vi "transport char run_subvi_08_24_12a_JW.vi"(0 "VISA session":refnum<visa-resource-name>="GPIB0::17::INSTR", 5 "Var1 sweep settings":T4={"start"=0.0, "stop"=-60.0, "step (linear only)"=-1.0, "sweep spacing (linear: 0)"=0, "sweep mode"=FALSE, "compliance (V)"=100.0, "compliance (A)"=0.001} {"compliance (A)" format="%^.2e"; "compliance (V)" format="%.2f"; "sweep spacing (linear: 0)" items=["linear", "log 10", "log 25", "log 50"]; "step (linear only)" format="%.2f"; "stop" format="%.2f"; "start" format="%.2f"}, 7 "Var2 step settings":T3={"compliance (A)"=0.001, "compliance (V)"=100.0, "start"=0.0, "total points"=7, "step"=-10.0} {"step" format="%.2f"; "start" format="%.2f"; "compliance (V)" format="%.2f"; "compliance (A)" format="%^.2e"}, 9 "integration time":u32(slide) scale=0.0..2.0, 11 "Path":path, 13 "Sample Properties:":T1 {"Date Created" format="%<%Y/%m/%d>T"}) -> (6 "graphic display":cluster{"trace":dbl[], "trace":dbl[]}(graph), 8 "Graph Cluster":cluster{"Transport":cluster{dbl[], dbl[]}[]}, 15 "error?":errorcluster)   [LabVIEW 2011]
uses:
  <vilib>/Utility/file.llb/Write To Spreadsheet File (DBL).vi
panel:
  in  "Temp (K)":dbl=100.0 format="%^.2e"
  in  "MAXIMUM":ext format="%.2e"
  in  "MINIMUM":ext=-1e-05 format="%_2e"
  out "graphic display 2":cluster{"trace":dbl[], "trace":dbl[]}(graph)
  in  "Y1 axis":string="Id"
  in  "Y2 axis settings":T2={"Y2 axis on/off"=FALSE, "MINIMUM"=-1e-07, "MAXIMUM"=1e-07, "Variable name"="", "LIN or LOG axis"=""} {"MAXIMUM" format="%.2e"; "MINIMUM" format="%.2e"}
  in  "wait time parameter":dbl=1.0
  in  "Value (Either V or A) 4":dbl
  in  "Value (Either V or A) 3":dbl
  in  "Value (Either V or A) 2":dbl
  in  "Value (V or A)":dbl
  in  "compliance (A)":dbl=0.001 format="%^.2e"
  in  "compliance (V)":dbl=100.0 format="%^.2e"
  in  "Iname":string="Is"
  in  "Vname":string="Vs"
  in  "Function":u16(ring)=4 items=["disabled", "Var1", "Var2", "Var1'", "Constant"]
  in  "Mode":u16(ring)=4 items=["V", "I", "VPulse", "IPulse", "Common"]
  in  "Iname 4":string="I4"
  in  "Vname 4":string="V4"
  in  "Function 4":u16(ring)=4 items=["disabled", "Var1", "Var2", "Var1'", "Constant"]
  in  "Mode 4":u16(ring) items=["V", "I", "VPulse", "IPulse", "Common"]
  in  "Iname 3":string="Ig"
  in  "Vname 3":string="Vg"
  in  "Function 3":u16(ring)=2 items=["disabled", "Var1", "Var2", "Var1'", "Constant"]
  in  "Mode 3":u16(ring) items=["V", "I", "VPulse", "IPulse", "Common"]
  in  "Iname 2":string="Id"
  in  "Vname 2":string="Vd"
  in  "Function 2":u16(ring)=1 items=["disabled", "Var1", "Var2", "Var1'", "Constant"]
  in  "Mode 2":u16(ring) items=["V", "I", "VPulse", "IPulse", "Common"]
  in  "reset":bool=TRUE
  # "SMU1"
  # "SMU2"
  # "SMU3"
  # "SMU4"
  # "%"
  # "nm"
  # "Device Properties:"
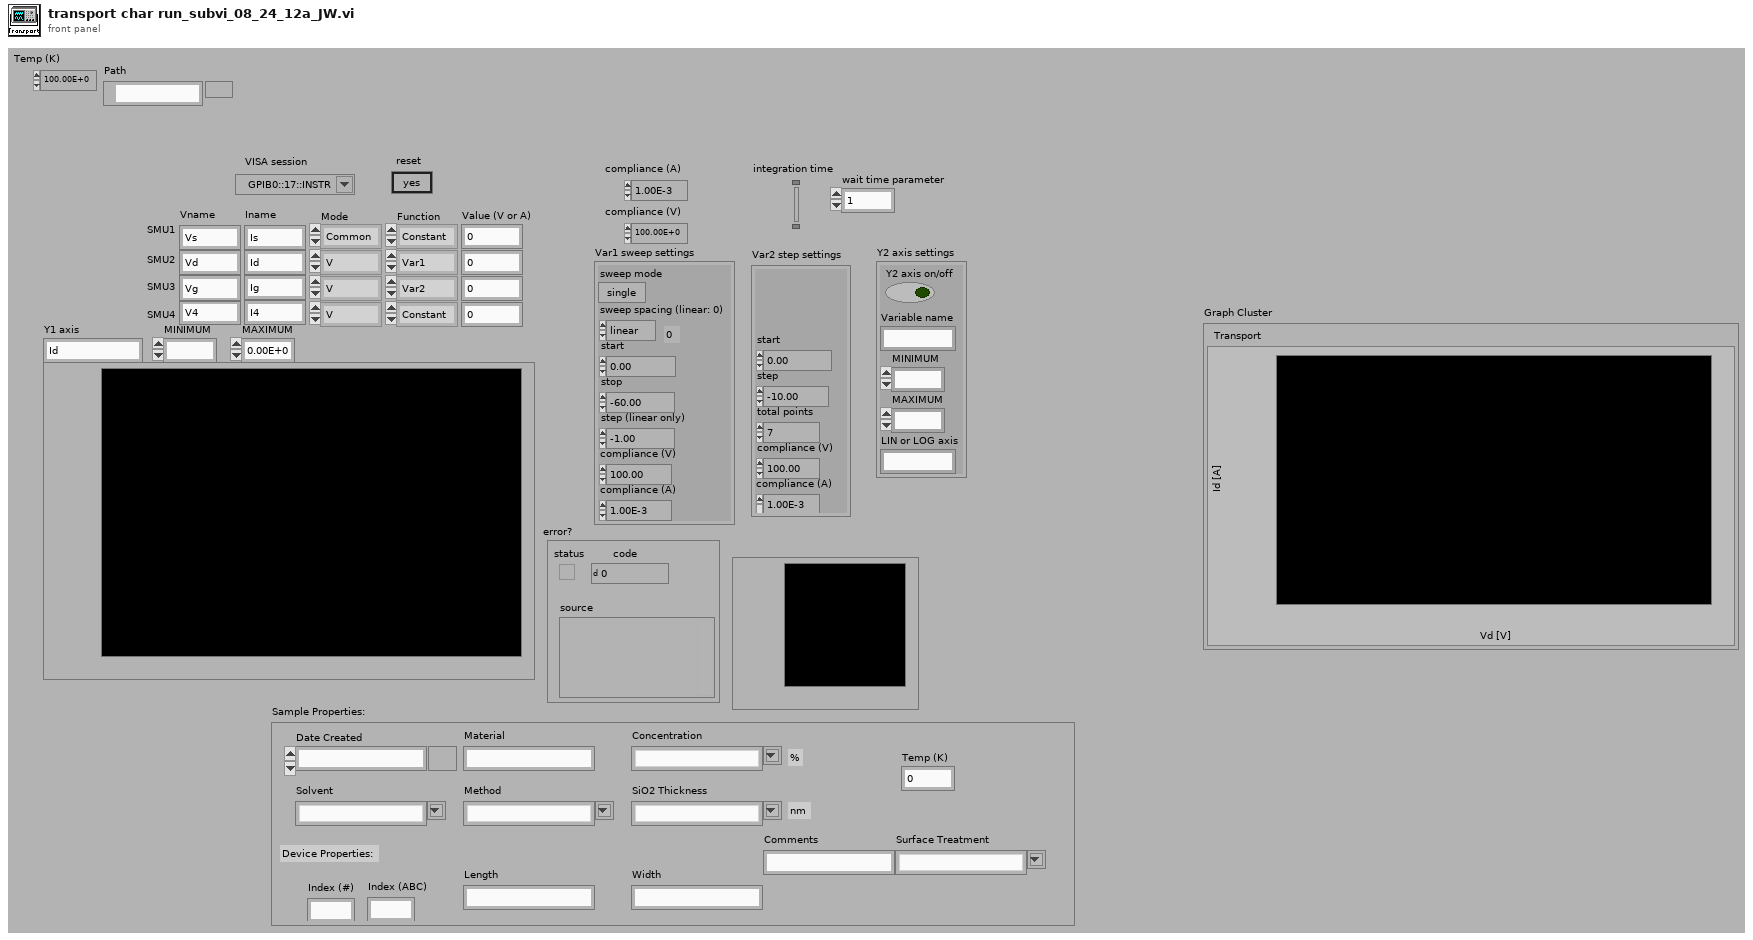
[diagram p1: front panel]
types:
  T1 = cluster{"Date Created":timestamp, "Material":string, "Solvent":string, "Concentration":string, "Method":string, "SiO2 Thickness":string, "Index (#)":string, "Index (ABC)":string, "Length":string, "Width":string, "Surface Treatment":string, "Comments":string, "Temp (K)":dbl}
  T2 = cluster{"Y2 axis on/off":bool, "MINIMUM":ext, "MAXIMUM":ext, "Variable name":string, "LIN or LOG axis":string}
  T3 = cluster{"compliance (A)":dbl, "compliance (V)":dbl, "start":dbl, "total points":u16, "step":dbl}
  T4 = cluster{"start":dbl, "stop":dbl, "step (linear only)":dbl, "sweep spacing (linear: 0)":u16, "sweep mode":bool, "compliance (V)":dbl, "compliance (A)":dbl}
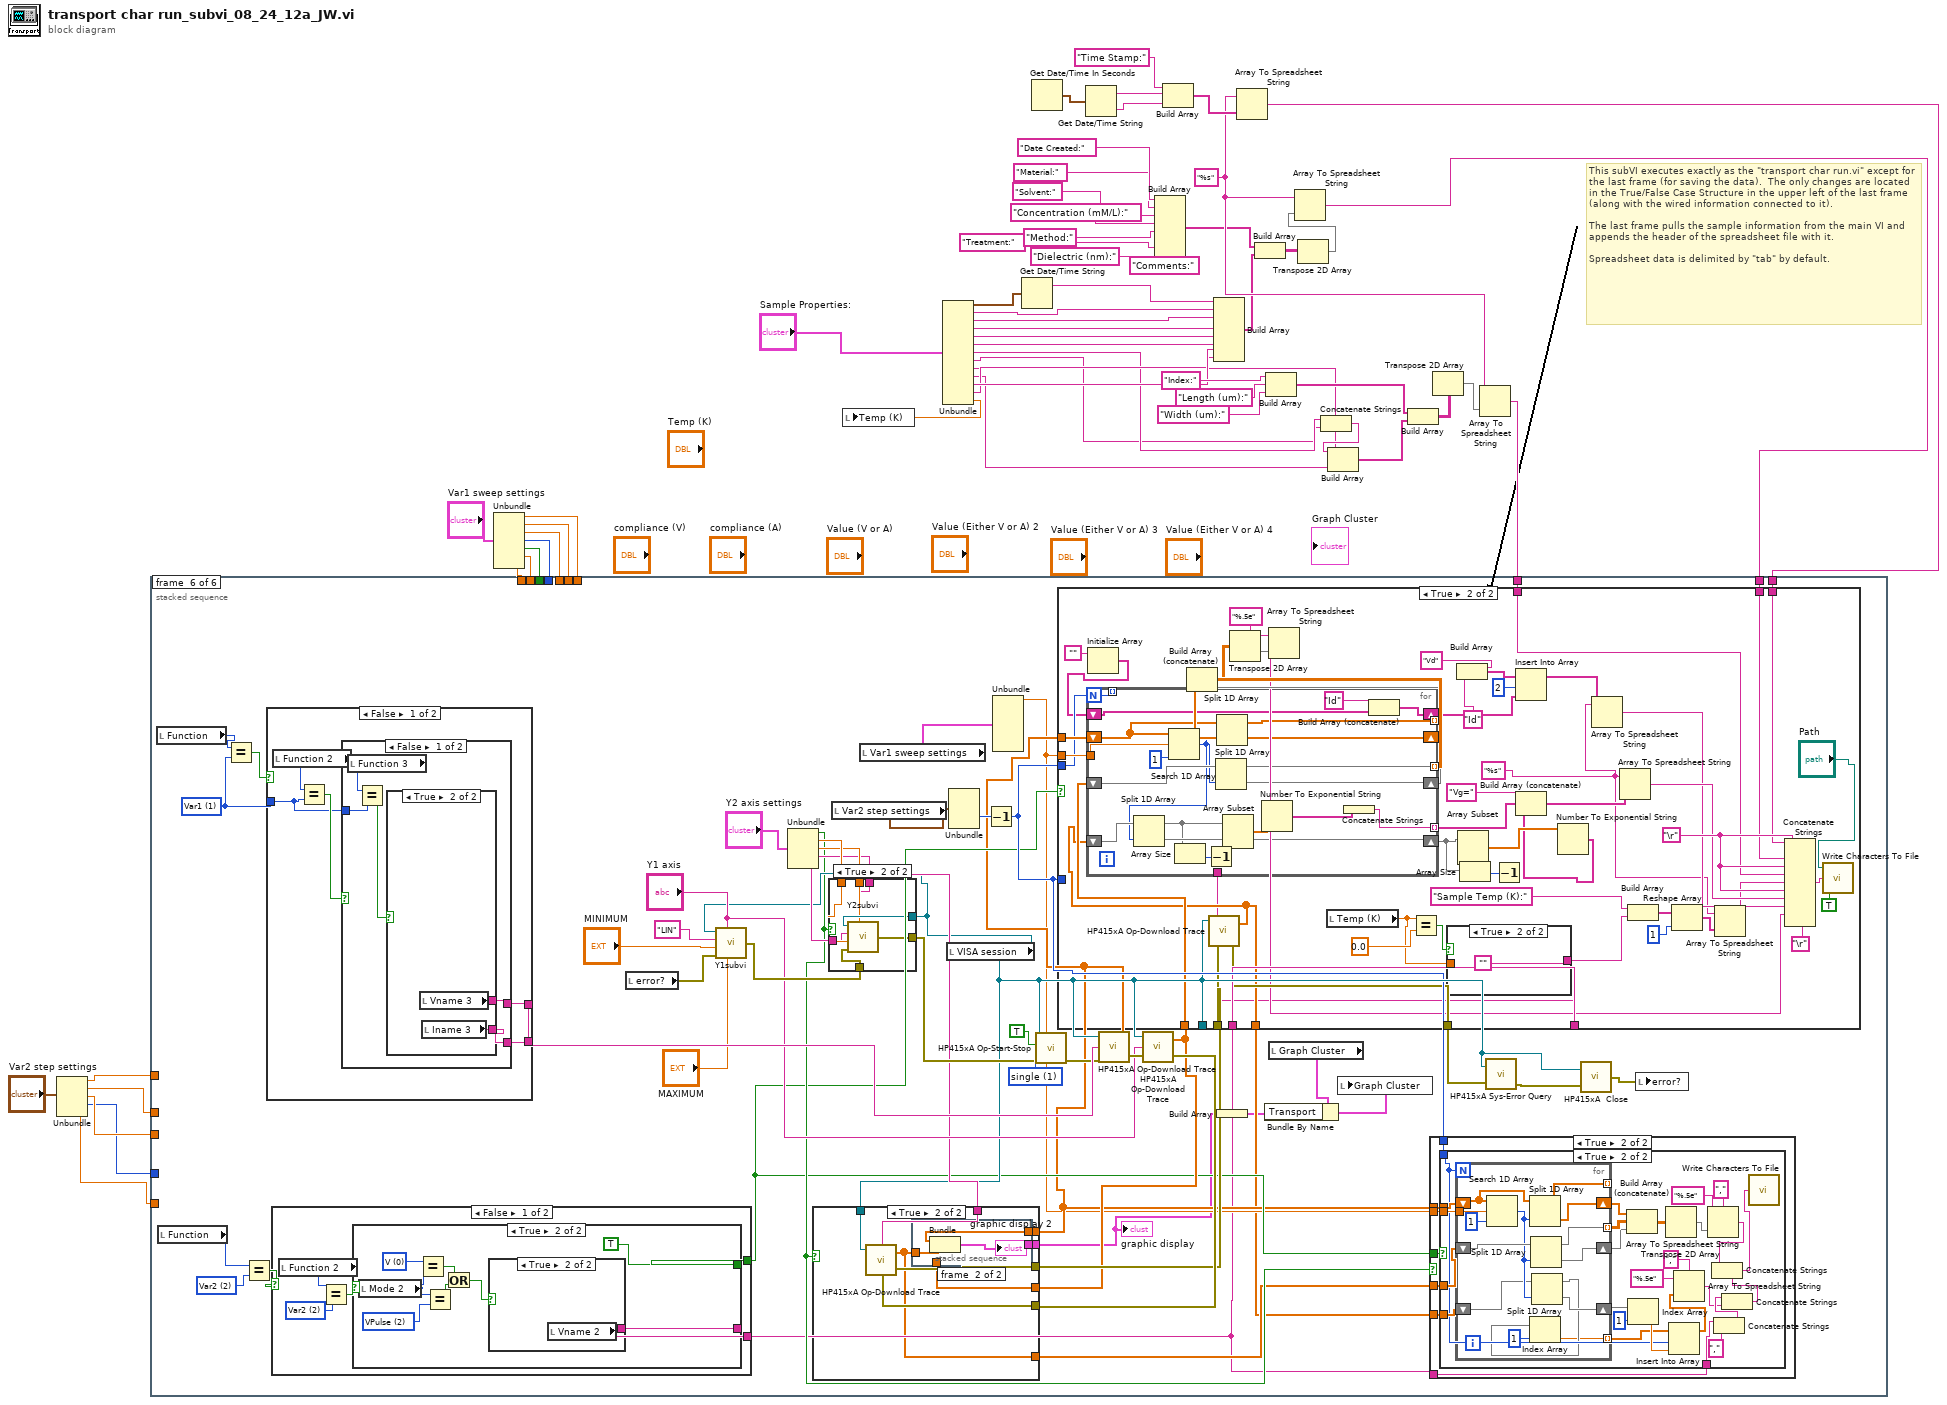
[diagram p0: block diagram]
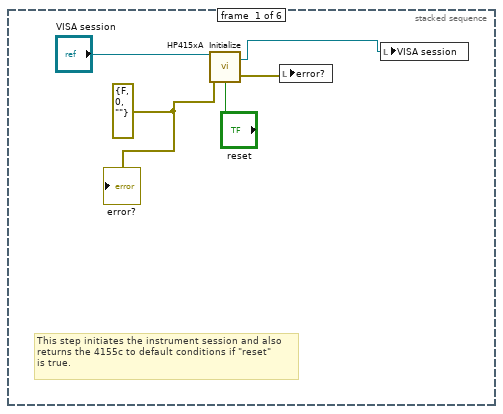
[diagram p2: hidden frame]
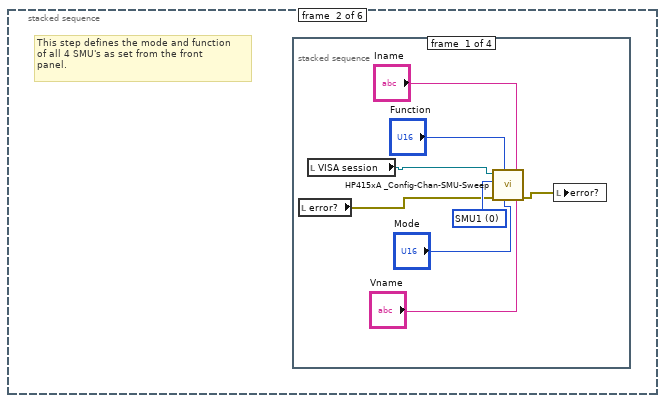
[diagram p3: hidden frame]
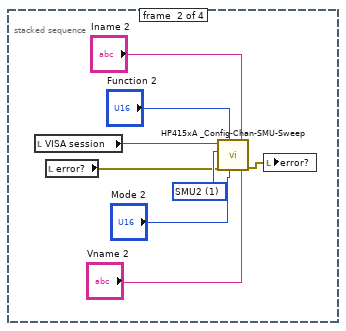
[diagram p4: hidden frame]
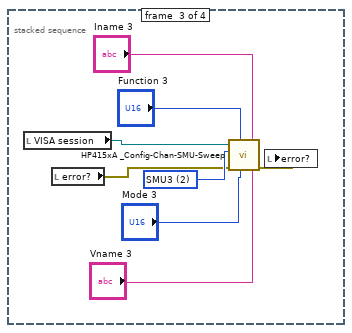
[diagram p5: hidden frame]
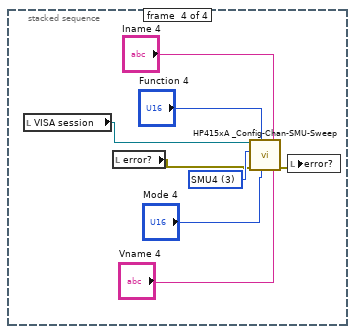
[diagram p6: hidden frame]
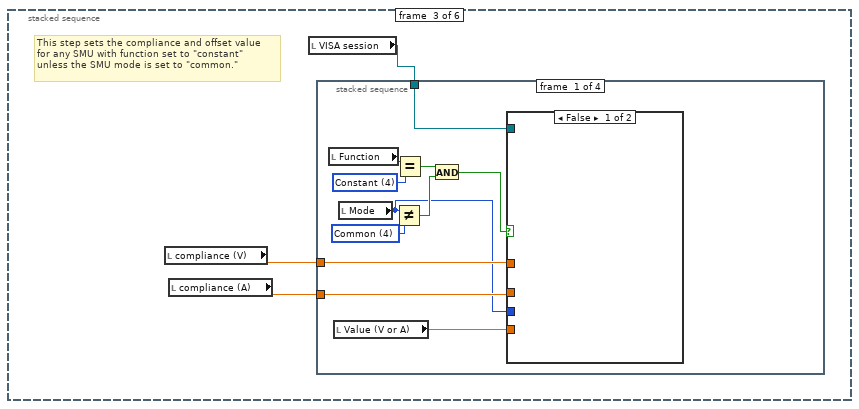
[diagram p7: hidden frame]
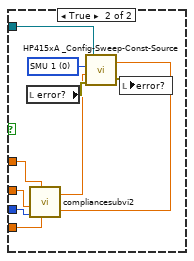
[diagram p8: hidden frame]
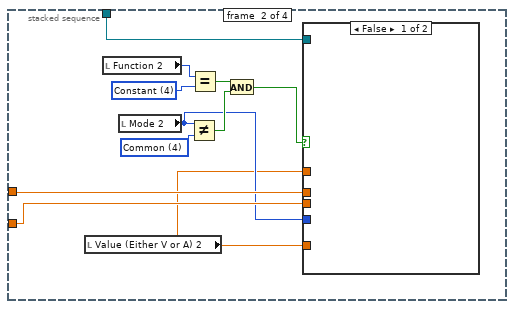
[diagram p9: hidden frame]
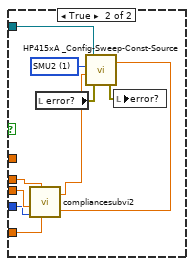
[diagram p10: hidden frame]
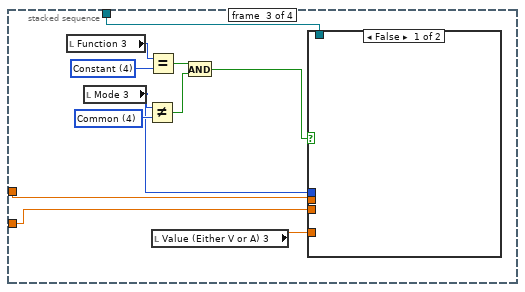
[diagram p11: hidden frame]
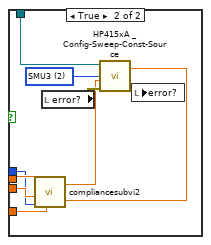
[diagram p12: hidden frame]
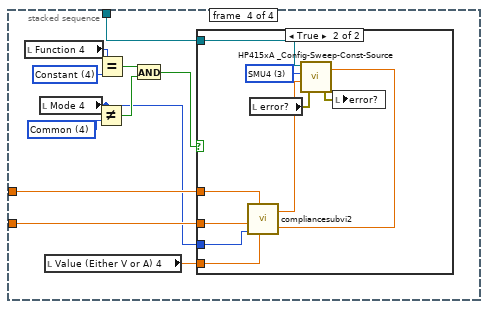
[diagram p13: hidden frame]
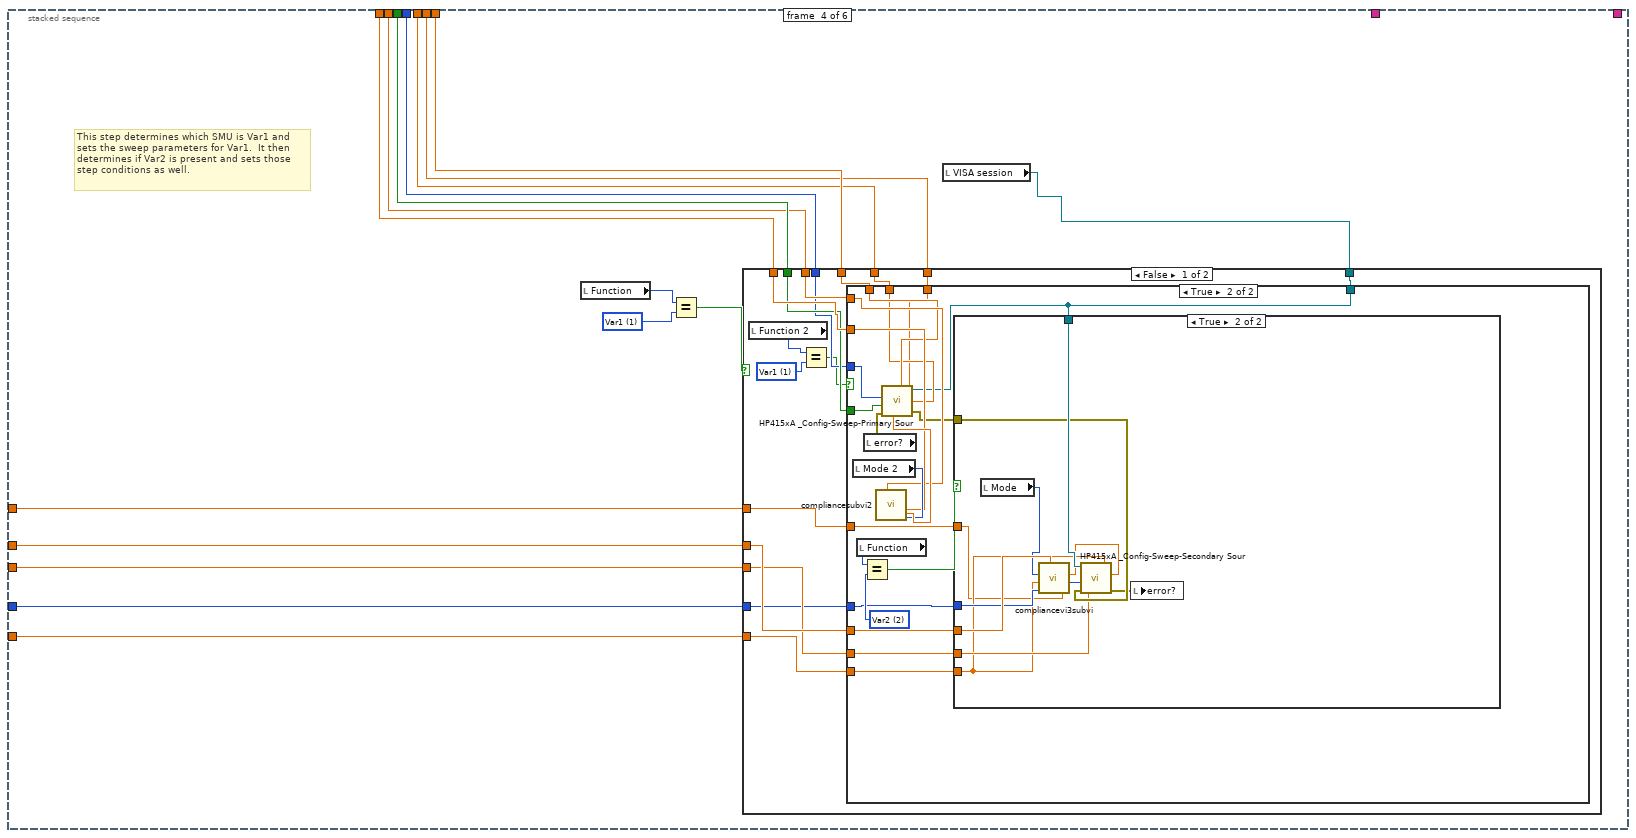
[diagram p15: hidden frame]
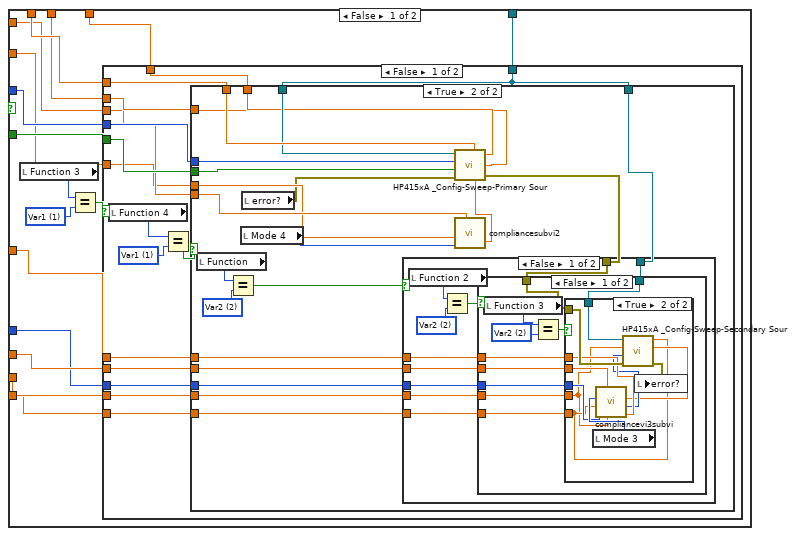
[diagram p16: hidden frame]
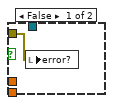
[diagram p18: hidden frame]
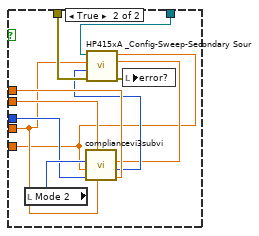
[diagram p19: hidden frame]
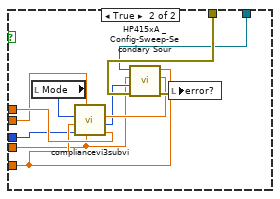
[diagram p20: hidden frame]
diagram:
  w32 = "%s"
  # "This subVI executes exactly as the \"transport char run.vi\" except for the last frame (for saving the data).  The only changes are located in the True/False Case Structure in the upper left of the last frame (along with the wired information connected to it). \n\nThe last frame pulls the sample information from the main VI and appends the header of the spreadsheet file with it.\n\nSpreadsheet data is delimited by \"tab\" by default."
  n1 = Unbundle("Var2 step settings") -> ("compliance (A)"=w49:dbl, "compliance (V)"=w48:dbl, "start"=w47:dbl, "total points"=w46:u16, "step"=w45:dbl)
  n2 = Unbundle("Var1 sweep settings") -> ("start"=w57:dbl, "stop"=w56:dbl, "step (linear only)"=w55:dbl, "sweep spacing (linear: 0)"=w54:u16, "sweep mode"=w53:bool, "compliance (V)"=w52:dbl, "compliance (A)"=w51:dbl)
  n3 = Unbundle("Sample Properties:") -> ("Date Created"=w16:timestamp, "Material"=w15:string, "Solvent"=w11:string, "Concentration"=w9:string, "Method"=w14:string, "SiO2 Thickness"=w10:string, "Index (#)"=w6:string, "Index (ABC)"=w5:string, "Length"=w3:string, "Width"=w2:string, "Surface Treatment"=w8:string, "Comments"=w7:string, "Temp (K)"=w1:dbl)
  n4 = local write "Temp (K)"(w1) -> ()
  n5 = Get Date/Time String(seconds (now)=w16) -> (date string=w44:string)  [unwired: 2 in, 1 out]
  n6 = Get Date/Time In Seconds() -> (seconds since 1Jan1904=w39:timestamp)
  n7 = Get Date/Time String(seconds (now)=w39) -> (date string=w38:string, time string=w37:string)  [unwired: 2 in]
  n8 = Build Array("Date Created:", "Material:", "Solvent:", "Concentration (mM/L):", "Method:", "Dielectric (nm):", "Treatment:", "Comments:") -> (w25:string[])
  n9 = Build Array("Time Stamp:", w38, w37) -> (w36:string[])
  n10 = Build Array(w44, w15, w11, w9, w14, w10, w8, w7) -> (w24:string[])
  n11 = Array To Spreadsheet String(array=w36, 3:w32) -> (spreadsheet string=w31:string)  [unwired: 1 in]
  n12 = Build Array(w25, w24) -> (w23:string[][])
  n13 = Build Array("Index:", "Length (um):", "Width (um):") -> (w21:string[])
  n14 = Transpose 2D Array(2D array=w23) -> (transposed array=w22:string[][])
  n15 = Array To Spreadsheet String(array=w22, 3:w32) -> (spreadsheet string=w30:string)  [unwired: 1 in]
  n16 = Concatenate Strings(w6, w5) -> (w4:string)
  n17 = Build Array(w4, w3, w2) -> (w20:string[])
  n18 = Build Array(w21, w20) -> (w19:string[][])
  n19 = Transpose 2D Array(2D array=w19) -> (transposed array=w18:string[][])
  n20 = Array To Spreadsheet String(array=w18, 3:w32) -> (spreadsheet string=w29:string)  [unwired: 1 in]
  n21 = stacked-sequence {
    tunnel: w57 -> [_ _ _ w194 _ _]
    tunnel: w56 -> [_ _ _ w193 _ _]
    tunnel: w55 -> [_ _ _ w192 _ _]
    tunnel: w54 -> [_ _ _ w191 _ _]
    tunnel: w53 -> [_ _ _ w190 _ _]
    tunnel: w52 -> [_ _ _ w189 _ _]
    tunnel: w51 -> [_ _ _ w188 _ _]
    tunnel: w49 -> [_ _ _ w187 _ _]
    tunnel: w48 -> [_ _ _ w186 _ _]
    tunnel: w47 -> [_ _ _ w185 _ _]
    tunnel: w46 -> [_ _ _ w184 _ _]
    tunnel: w45 -> [_ _ _ w183 _ _]
    tunnel: w31 -> [_ _ _ _ _ w555]
    tunnel: w30 -> [_ _ _ _ _ w554]
    tunnel: w29 -> [_ _ _ _ _ w553]
    frame #0 {
      w62 = errorcluster {"status"=FALSE, "code"=0, "source"=""} ("error out")
      # "This step initiates the instrument session and also\nreturns the 4155c to default conditions if \"reset\"\nis true."
      n22 = call "HP415xA  Initialize.vi"("instrument descriptor"="VISA session", "reset"="reset", "error in (no error)"=w62) -> ("VISA session"=w59:refnum<visa-resource-name>, "error out"=w61:errorcluster)  [unwired: 2 in]
      n23 = local write "error?"(w61) -> ()
      n24 = local write "VISA session"(w59) -> ()
      "error?" <- w62
    }
    frame #1 {
      # "This step defines the mode and function\nof all 4 SMU's as set from the front\npanel."
      n25 = stacked-sequence {
        frame #0 {
          w71 = u32 0 items=["SMU1  ", "SMU2  ", "SMU3  ", "SMU4  ", "SMU5  ", "SMU6  "] ("unit to configure")
          n26 = local read "error?"() -> (w66:errorcluster)
          n27 = local read "VISA session"() -> (w64:refnum<visa-resource-name>)
          n28 = call "HP415xA _Config-Chan-SMU-Sweep.vi"("V name (max 6 chars)"="Vname", "I name (max 6 chars)"="Iname", "mode"="Mode", "function"="Function", "error in (no error)"=w66, "unit to configure"=w71, "VISA session"=w64) -> ("error out"=w65:errorcluster)  [unwired: 2 in]
          n29 = local write "error?"(w65) -> ()
        }
        frame #1 {
          w75 = u32 1 items=["SMU1  ", "SMU2  ", "SMU3  ", "SMU4  ", "SMU5  ", "SMU6  "] ("unit to configure")
          n30 = local read "VISA session"() -> (w72:refnum<visa-resource-name>)
          n31 = local read "error?"() -> (w73:errorcluster)
          n32 = call "HP415xA _Config-Chan-SMU-Sweep.vi"("V name (max 6 chars)"="Vname 2", "I name (max 6 chars)"="Iname 2", "mode"="Mode 2", "function"="Function 2", "error in (no error)"=w73, "unit to configure"=w75, "VISA session"=w72) -> ("error out"=w74:errorcluster)  [unwired: 2 in]
          n33 = local write "error?"(w74) -> ()
        }
        frame #2 {
          w83 = u32 2 items=["SMU1  ", "SMU2  ", "SMU3  ", "SMU4  ", "SMU5  ", "SMU6  "] ("unit to configure")
          n34 = local read "VISA session"() -> (w80:refnum<visa-resource-name>)
          n35 = local read "error?"() -> (w81:errorcluster)
          n36 = call "HP415xA _Config-Chan-SMU-Sweep.vi"("V name (max 6 chars)"="Vname 3", "I name (max 6 chars)"="Iname 3", "mode"="Mode 3", "function"="Function 3", "error in (no error)"=w81, "unit to configure"=w83, "VISA session"=w80) -> ("error out"=w82:errorcluster)  [unwired: 2 in]
          n37 = local write "error?"(w82) -> ()
        }
        frame #3 {
          w91 = u32 3 items=["SMU1  ", "SMU2  ", "SMU3  ", "SMU4  ", "SMU5  ", "SMU6  "] ("unit to configure")
          n38 = local read "VISA session"() -> (w88:refnum<visa-resource-name>)
          n39 = local read "error?"() -> (w90:errorcluster)
          n40 = call "HP415xA _Config-Chan-SMU-Sweep.vi"("V name (max 6 chars)"="Vname 4", "I name (max 6 chars)"="Iname 4", "mode"="Mode 4", "function"="Function 4", "error in (no error)"=w90, "unit to configure"=w91, "VISA session"=w88) -> ("error out"=w89:errorcluster)  [unwired: 2 in]
          n41 = local write "error?"(w89) -> ()
        }
      }
    }
    frame #2 {
      # "This step sets the compliance and offset value\nfor any SMU with function set to \"constant\"\nunless the SMU mode is set to \"common.\""
      n42 = local read "compliance (V)"() -> (w97:dbl)
      n43 = local read "compliance (A)"() -> (w98:dbl)
      n44 = local read "VISA session"() -> (w96:refnum<visa-resource-name>)
      n45 = stacked-sequence {
        tunnel: w96 -> [w107 w127 w146 w166]
        tunnel: w98 -> [w101 w123 w144 w164]
        tunnel: w97 -> [w100 w122 w143 w165]
        frame #0 {
          w105 = u16 4 items=["V", "I", "VPulse", "IPulse", "Common"] ("Mode")
          w109 = u16 4 items=["disabled", "Var1", "Var2", "Var1'", "Constant"] ("Function")
          n46 = local read "Function"() -> (w108:u16)
          n47 = local read "Value (V or A)"() -> (w102:dbl)
          n48 = local read "Mode"() -> (w99:u16)
          n49 = Not Equal?(x=w99, y=w105) -> (x != y?=w104:bool)
          n50 = Equal?(x=w108, y=w109) -> (x = y?=w106:bool)
          n51 = And(x=w106, y=w104) -> (x .and. y?=w103:bool)
          n52 = case shown="False" w103 {
            tunnel: w107 -> [_ w119]
            tunnel: w100 -> [_ w115]
            tunnel: w101 -> [_ w114]
            tunnel: w102 -> [_ w111]
            tunnel: w99 -> [_ w112]
            frame False {
            }
            frame True {
              w118 = u16 0 items=["SMU 1", "SMU2", "SMU3", "SMU4", "SMU5", "SMU6", "VSU1", "VSU2"] ("unit (SMU1:0)")
              n53 = local read "error?"() -> (w117:errorcluster)
              n54 = call "compliancesubvi2.vi"("Value1"=w111, "compliance (V)"=w115, "Mode"=w112, "compliance (A)"=w114) -> ("compliance"=w113:dbl, "constant"=w110:dbl)  [unwired: 2 in]
              n55 = call "HP415xA _Config-Sweep-Const-Source.vi"("compliance (SMUs only)"=w113, "error in (no error)"=w117, "source (V or A)"=w110, "unit (SMU1:0)"=w118, "VISA session"=w119) -> ("error out"=w116:errorcluster)
              n56 = local write "error?"(w116) -> ()
            }
          }
        }
        frame #1 {
          w124 = u16 4 items=["V", "I", "VPulse", "IPulse", "Common"] ("Mode 2")
          w125 = u16 4 items=["disabled", "Var1", "Var2", "Var1'", "Constant"] ("Function 2")
          n57 = local read "Value (Either V or A) 2"() -> (w120:dbl)
          n58 = local read "Function 2"() -> (w126:u16)
          n59 = local read "Mode 2"() -> (w121:u16)
          n60 = Not Equal?(x=w121, y=w124) -> (x != y?=w129:bool)
          n61 = Equal?(x=w126, y=w125) -> (x = y?=w130:bool)
          n62 = And(x=w130, y=w129) -> (x .and. y?=w128:bool)
          n63 = case shown="False" w128 {
            tunnel: w127 -> [_ w140]
            tunnel: w122 -> [_ w138]
            tunnel: w123 -> [_ w137]
            tunnel: w120 -> [_ _]
            tunnel: w121 -> [_ w133]
            tunnel: w120 -> [_ w132]
            frame False {
            }
            frame True {
              w139 = u16 1 items=["SMU 1", "SMU2", "SMU3", "SMU4", "SMU5", "SMU6", "VSU1", "VSU2"] ("unit (SMU1:0)")
              n64 = call "compliancesubvi2.vi"("Value1"=w132, "compliance (V)"=w138, "Mode"=w133, "compliance (A)"=w137) -> ("compliance"=w136:dbl, "constant"=w131:dbl)  [unwired: 2 in]
              n65 = local read "error?"() -> (w135:errorcluster)
              n66 = call "HP415xA _Config-Sweep-Const-Source.vi"("compliance (SMUs only)"=w136, "error in (no error)"=w135, "source (V or A)"=w131, "unit (SMU1:0)"=w139, "VISA session"=w140) -> ("error out"=w134:errorcluster)
              n67 = local write "error?"(w134) -> ()
            }
          }
        }
        frame #2 {
          w148 = u16 4 items=["V", "I", "VPulse", "IPulse", "Common"] ("Mode 2")
          w149 = u16 4 items=["disabled", "Var1", "Var2", "Var1'", "Constant"] ("Function 2")
          n68 = local read "Function 3"() -> (w147:u16)
          n69 = local read "Mode 3"() -> (w142:u16)
          n70 = Not Equal?(x=w142, y=w148) -> (x != y?=w150:bool)
          n71 = Equal?(x=w147, y=w149) -> (x = y?=w151:bool)
          n72 = local read "Value (Either V or A) 3"() -> (w145:dbl)
          n73 = And(x=w151, y=w150) -> (x .and. y?=w141:bool)
          n74 = case shown="False" w141 {
            tunnel: w146 -> [_ w159]
            tunnel: w145 -> [_ w153]
            tunnel: w144 -> [_ w156]
            tunnel: w143 -> [_ w155]
            tunnel: w142 -> [_ w154]
            frame False {
            }
            frame True {
              w158 = u16 2 items=["SMU 1", "SMU2", "SMU3", "SMU4", "SMU5", "SMU6", "VSU1", "VSU2"] ("unit (SMU1:0)")
              n75 = call "compliancesubvi2.vi"("Value1"=w153, "compliance (V)"=w155, "Mode"=w154, "compliance (A)"=w156) -> ("compliance"=w157:dbl, "constant"=w152:dbl)  [unwired: 2 in]
              n76 = local read "error?"() -> (w161:errorcluster)
              n77 = call "HP415xA _Config-Sweep-Const-Source.vi"("compliance (SMUs only)"=w157, "error in (no error)"=w161, "source (V or A)"=w152, "unit (SMU1:0)"=w158, "VISA session"=w159) -> ("error out"=w160:errorcluster)
              n78 = local write "error?"(w160) -> ()
            }
          }
        }
        frame #3 {
          w168 = u16 4 items=["V", "I", "VPulse", "IPulse", "Common"] ("Mode 4")
          w169 = u16 4 items=["disabled", "Var1", "Var2", "Var1'", "Constant"] ("Function 4")
          n79 = local read "Function 4"() -> (w170:u16)
          n80 = local read "Mode 4"() -> (w163:u16)
          n81 = local read "Value (Either V or A) 4"() -> (w162:dbl)
          n82 = Not Equal?(x=w163, y=w168) -> (x != y?=w171:bool)
          n83 = Equal?(x=w170, y=w169) -> (x = y?=w172:bool)
          n84 = And(x=w172, y=w171) -> (x .and. y?=w167:bool)
          n85 = case shown="True" w167 {
            tunnel: w166 -> [_ w181]
            tunnel: w165 -> [_ w177]
            tunnel: w164 -> [_ w178]
            tunnel: w163 -> [_ w176]
            tunnel: w162 -> [_ w175]
            frame False {
            }
            frame True {
              w182 = u16 3 items=["SMU 1", "SMU2", "SMU3", "SMU4", "SMU5", "SMU6", "VSU1", "VSU2"] ("unit (SMU1:0)")
              n86 = call "compliancesubvi2.vi"("Value1"=w175, "compliance (V)"=w177, "Mode"=w176, "compliance (A)"=w178) -> ("compliance"=w174:dbl, "constant"=w173:dbl)  [unwired: 2 in]
              n87 = local read "error?"() -> (w180:errorcluster)
              n88 = call "HP415xA _Config-Sweep-Const-Source.vi"("compliance (SMUs only)"=w174, "error in (no error)"=w180, "source (V or A)"=w173, "unit (SMU1:0)"=w182, "VISA session"=w181) -> ("error out"=w179:errorcluster)
              n89 = local write "error?"(w179) -> ()
            }
          }
        }
      }
    }
    frame #3 {
      w198 = u16 1 items=["disabled", "Var1", "Var2", "Var1'", "Constant"] ("Function")
      # "This step determines which SMU is Var1 and\nsets the sweep parameters for Var1.  It then\ndetermines if Var2 is present and sets those\nstep conditions as well."
      n90 = local read "Function"() -> (w197:u16)
      n91 = Equal?(x=w197, y=w198) -> (x = y?=w196:bool)
      n92 = local read "VISA session"() -> (w195:refnum<visa-resource-name>)
      n93 = case shown="False" w196 {
        tunnel: w189 -> [w211 w487]
        tunnel: w188 -> [w212 w486]
        tunnel: w191 -> [w209 w485]
        tunnel: w190 -> [w210 w484]
        tunnel: w192 -> [w206 w483]
        tunnel: w193 -> [w205 w482]
        tunnel: w194 -> [w207 w481]
        tunnel: w195 -> [w208 w470]
        tunnel: w187 -> [w203 w476]
        tunnel: w186 -> [w202 w475]
        tunnel: w185 -> [w201 w474]
        tunnel: w184 -> [w200 w473]
        tunnel: w183 -> [w199 w472]
        frame False {
          w214 = u16 1 items=["disabled", "Var1", "Var2", "Var1'", "Constant"] ("Function")
          n94 = local read "Function 2"() -> (w213:u16)
          n95 = Equal?(x=w213, y=w214) -> (x = y?=w204:bool)
          n96 = case shown="True" w204 {
            tunnel: w212 -> [w220 w413]
            tunnel: w211 -> [w221 w412]
            tunnel: w210 -> [w222 w411]
            tunnel: w209 -> [w223 w410]
            tunnel: w208 -> [w227 w399]
            tunnel: w207 -> [w226 w409]
            tunnel: w206 -> [w224 w408]
            tunnel: w205 -> [w225 w407]
            tunnel: w203 -> [w219 w402]
            tunnel: w202 -> [w218 w401]
            tunnel: w201 -> [w216 w400]
            tunnel: w200 -> [w217 w397]
            tunnel: w199 -> [w215 w396]
            frame False {
              w230 = u16 1 items=["disabled", "Var1", "Var2", "Var1'", "Constant"] ("Function")
              n97 = local read "Function 3"() -> (w229:u16)
              n98 = Equal?(x=w229, y=w230) -> (x = y?=w228:bool)
              n99 = case shown="False" w228 {
                tunnel: w227 -> [w231 w324]
                tunnel: w226 -> [w243 w341]
                tunnel: w225 -> [w240 w340]
                tunnel: w224 -> [w239 w339]
                tunnel: w223 -> [w242 w338]
                tunnel: w222 -> [w241 w337]
                tunnel: w221 -> [w238 w336]
                tunnel: w220 -> [w237 w335]
                tunnel: w219 -> [w236 w328]
                tunnel: w218 -> [w235 w327]
                tunnel: w217 -> [w234 w326]
                tunnel: w216 -> [w233 w323]
                tunnel: w215 -> [w232 w322]
                frame False {
                  w246 = u16 1 items=["disabled", "Var1", "Var2", "Var1'", "Constant"] ("Function")
                  n100 = local read "Function 4"() -> (w245:u16)
                  n101 = Equal?(x=w245, y=w246) -> (x = y?=w244:bool)
                  n102 = case shown="True" w244 {
                    tunnel: w243 -> [_ w265]
                    tunnel: w231 -> [_ w264]
                    tunnel: w242 -> [_ w263]
                    tunnel: w241 -> [_ w262]
                    tunnel: w240 -> [_ w261]
                    tunnel: w239 -> [_ w260]
                    tunnel: w238 -> [_ w259]
                    tunnel: w237 -> [_ w258]
                    tunnel: w236 -> [_ w253]
                    tunnel: w235 -> [_ w252]
                    tunnel: w234 -> [_ w251]
                    tunnel: w233 -> [_ w250]
                    tunnel: w232 -> [_ w249]
                    tunnel: w231 -> [_ w247]
                    frame False {
                    }
                    frame True {
                      w256 = u16 2 items=["disabled", "Var1", "Var2", "Var1'", "Constant"] ("Function")
                      n103 = local read "Function"() -> (w255:u16)
                      n104 = Equal?(x=w255, y=w256) -> (x = y?=w254:bool)
                      n105 = local read "Mode 4"() -> (w267:u16)
                      n106 = local read "error?"() -> (w257:errorcluster)
                      n107 = call "compliancesubvi2.vi"("compliance (V)"=w259, "Mode"=w267, "compliance (A)"=w258) -> ("compliance"=w266:dbl)  [unwired: 3 in, 1 out]
                      n108 = call "HP415xA _Config-Sweep-Primary Sour.vi"("step (linear only)"=w260, "stop"=w261, "start"=w265, "compliance"=w266, "error in (no error)"=w257, "sweep mode"=w262, "sweep spacing (linear: 0)"=w263, "VISA session"=w264) -> ("error out"=w248:errorcluster)  [unwired: 2 in]
                      n109 = case shown="False" w254 {
                        tunnel: w253 -> [w274 w317]
                        tunnel: w252 -> [w273 w312]
                        tunnel: w251 -> [w272 w311]
                        tunnel: w250 -> [w271 w313]
                        tunnel: w249 -> [w270 w316]
                        tunnel: w248 -> [w269 w319]
                        tunnel: w247 -> [w268 w318]
                        frame False {
                          w277 = u16 2 items=["disabled", "Var1", "Var2", "Var1'", "Constant"] ("Function")
                          n110 = local read "Function 2"() -> (w276:u16)
                          n111 = Equal?(x=w276, y=w277) -> (x = y?=w275:bool)
                          n112 = case shown="False" w275 {
                            tunnel: w274 -> [w285 w305]
                            tunnel: w273 -> [w284 w306]
                            tunnel: w272 -> [w283 w304]
                            tunnel: w271 -> [w282 w302]
                            tunnel: w270 -> [w281 w300]
                            tunnel: w269 -> [w280 w310]
                            tunnel: w268 -> [w278 w309]
                            frame False {
                              w287 = u16 2 items=["disabled", "Var1", "Var2", "Var1'", "Constant"] ("Function")
                              n113 = local read "Function 3"() -> (w279:u16)
                              n114 = Equal?(x=w279, y=w287) -> (x = y?=w286:bool)
                              n115 = case shown="True" w286 {
                                tunnel: w285 -> [_ w293]
                                tunnel: w284 -> [_ w294]
                                tunnel: w283 -> [_ w295]
                                tunnel: w282 -> [_ w289]
                                tunnel: w281 -> [_ w290]
                                tunnel: w280 -> [w288 w299]
                                tunnel: w278 -> [_ w298]
                                frame False {
                                n116 = local write "error?"(w288) -> ()
                                }
                                frame True {
                                n117 = local read "Mode 3"() -> (w297:u16)
                                n118 = call "compliancevi3subvi.vi"("compliance (A)"=w293, "start"=w289, "compliance (V)"=w294, "total points"=w295, "step"=w290, "Mode"=w297) -> ("total points 2"=w292:u16, "compliance"=w291:dbl)  [unwired: 1 in, 1 out]
                                n119 = call "HP415xA _Config-Sweep-Secondary Sour.vi"("compliance"=w291, "step"=w290, "error in (no error)"=w299, "total points"=w292, "start"=w289, "VISA session"=w298) -> ("error out"=w296:errorcluster)  [unwired: 1 in]
                                n120 = local write "error?"(w296) -> ()
                                }
                              }
                            }
                            frame True {
                              n121 = local read "Mode 2"() -> (w308:u16)
                              n122 = call "compliancevi3subvi.vi"("compliance (A)"=w305, "start"=w302, "compliance (V)"=w306, "total points"=w304, "step"=w300, "Mode"=w308) -> ("total points 2"=w303:u16, "compliance"=w301:dbl)  [unwired: 1 in, 1 out]
                              n123 = call "HP415xA _Config-Sweep-Secondary Sour.vi"("compliance"=w301, "step"=w300, "error in (no error)"=w310, "total points"=w303, "start"=w302, "VISA session"=w309) -> ("error out"=w307:errorcluster)  [unwired: 1 in]
                              n124 = local write "error?"(w307) -> ()
                            }
                          }
                        }
                        frame True {
                          n125 = local read "Mode"() -> (w321:u16)
                          n126 = call "compliancevi3subvi.vi"("compliance (A)"=w317, "start"=w313, "compliance (V)"=w312, "total points"=w311, "step"=w316, "Mode"=w321) -> ("total points 2"=w314:u16, "compliance"=w315:dbl)  [unwired: 1 in, 1 out]
                          n127 = call "HP415xA _Config-Sweep-Secondary Sour.vi"("compliance"=w315, "step"=w316, "error in (no error)"=w319, "total points"=w314, "start"=w313, "VISA session"=w318) -> ("error out"=w320:errorcluster)  [unwired: 1 in]
                          n128 = local write "error?"(w320) -> ()
                        }
                      }
                    }
                  }
                }
                frame True {
                  w331 = u16 2 items=["disabled", "Var1", "Var2", "Var1'", "Constant"] ("Function")
                  n129 = local read "Function"() -> (w330:u16)
                  n130 = local read "Mode 3"() -> (w333:u16)
                  n131 = call "compliancesubvi2.vi"("compliance (V)"=w336, "Mode"=w333, "compliance (A)"=w335) -> ("compliance"=w334:dbl)  [unwired: 3 in, 1 out]
                  n132 = Equal?(x=w330, y=w331) -> (x = y?=w329:bool)
                  n133 = local read "error?"() -> (w332:errorcluster)
                  n134 = call "HP415xA _Config-Sweep-Primary Sour.vi"("step (linear only)"=w339, "stop"=w340, "start"=w341, "compliance"=w334, "error in (no error)"=w332, "sweep mode"=w337, "sweep spacing (linear: 0)"=w338, "VISA session"=w324) -> ("error out"=w325:errorcluster)  [unwired: 2 in]
                  n135 = case shown="False" w329 {
                    tunnel: w328 -> [w346 w391]
                    tunnel: w327 -> [w345 w390]
                    tunnel: w326 -> [w343 w389]
                    tunnel: w325 -> [w348 w394]
                    tunnel: w324 -> [w347 w393]
                    tunnel: w323 -> [w342 w386]
                    tunnel: w322 -> [w344 w385]
                    frame False {
                      w351 = u16 2 items=["disabled", "Var1", "Var2", "Var1'", "Constant"] ("Function")
                      n136 = local read "Function 2"() -> (w350:u16)
                      n137 = Equal?(x=w350, y=w351) -> (x = y?=w349:bool)
                      n138 = case shown="True" w349 {
                        tunnel: w348 -> [w358 w383]
                        tunnel: w347 -> [w357 w382]
                        tunnel: w346 -> [w356 w378]
                        tunnel: w345 -> [w355 w379]
                        tunnel: w344 -> [w352 w377]
                        tunnel: w343 -> [w354 w380]
                        tunnel: w342 -> [w353 w376]
                        frame False {
                          w361 = u16 2 items=["disabled", "Var1", "Var2", "Var1'", "Constant"] ("Function")
                          n139 = local read "Function 4"() -> (w360:u16)
                          n140 = Equal?(x=w360, y=w361) -> (x = y?=w359:bool)
                          n141 = case shown="True" w359 {
                            tunnel: w358 -> [w362 w371]
                            tunnel: w357 -> [_ w372]
                            tunnel: w356 -> [_ w368]
                            tunnel: w355 -> [_ w369]
                            tunnel: w354 -> [_ w367]
                            tunnel: w353 -> [_ w364]
                            tunnel: w352 -> [_ w363]
                            frame False {
                              n142 = local write "error?"(w362) -> ()
                            }
                            frame True {
                              n143 = local read "Mode 4"() -> (w373:u16)
                              n144 = call "compliancevi3subvi.vi"("compliance (A)"=w368, "start"=w364, "compliance (V)"=w369, "total points"=w367, "step"=w363, "Mode"=w373) -> ("total points 2"=w366:u16, "compliance"=w365:dbl)  [unwired: 1 in, 1 out]
                              n145 = call "HP415xA _Config-Sweep-Secondary Sour.vi"("compliance"=w365, "step"=w363, "error in (no error)"=w371, "total points"=w366, "start"=w364, "VISA session"=w372) -> ("error out"=w370:errorcluster)  [unwired: 1 in]
                              n146 = local write "error?"(w370) -> ()
                            }
                          }
                        }
                        frame True {
                          n147 = local read "Mode 2"() -> (w384:u16)
                          n148 = call "compliancevi3subvi.vi"("compliance (A)"=w378, "start"=w376, "compliance (V)"=w379, "total points"=w380, "step"=w377, "Mode"=w384) -> ("total points 2"=w375:u16, "compliance"=w374:dbl)  [unwired: 1 in, 1 out]
                          n149 = call "HP415xA _Config-Sweep-Secondary Sour.vi"("compliance"=w374, "step"=w377, "error in (no error)"=w383, "total points"=w375, "start"=w376, "VISA session"=w382) -> ("error out"=w381:errorcluster)  [unwired: 1 in]
                          n150 = local write "error?"(w381) -> ()
                        }
                      }
                    }
                    frame True {
                      n151 = local read "Mode"() -> (w395:u16)
                      n152 = call "compliancevi3subvi.vi"("compliance (A)"=w391, "start"=w386, "compliance (V)"=w390, "total points"=w389, "step"=w385, "Mode"=w395) -> ("total points 2"=w388:u16, "compliance"=w387:dbl)  [unwired: 1 in, 1 out]
                      n153 = call "HP415xA _Config-Sweep-Secondary Sour.vi"("compliance"=w387, "step"=w385, "error in (no error)"=w394, "total points"=w388, "start"=w386, "VISA session"=w393) -> ("error out"=w392:errorcluster)  [unwired: 1 in]
                      n154 = local write "error?"(w392) -> ()
                    }
                  }
                }
              }
            }
            frame True {
              w405 = u16 2 items=["disabled", "Var1", "Var2", "Var1'", "Constant"] ("Function")
              n155 = local read "Mode 2"() -> (w414:u16)
              n156 = local read "Function"() -> (w404:u16)
              n157 = Equal?(x=w404, y=w405) -> (x = y?=w403:bool)
              n158 = local read "error?"() -> (w406:errorcluster)
              n159 = call "compliancesubvi2.vi"("compliance (V)"=w412, "Mode"=w414, "compliance (A)"=w413) -> ("compliance"=w415:dbl)  [unwired: 3 in, 1 out]
              n160 = call "HP415xA _Config-Sweep-Primary Sour.vi"("step (linear only)"=w408, "stop"=w407, "start"=w409, "compliance"=w415, "error in (no error)"=w406, "sweep mode"=w411, "sweep spacing (linear: 0)"=w410, "VISA session"=w399) -> ("error out"=w398:errorcluster)  [unwired: 2 in]
              n161 = case shown="True" w403 {
                tunnel: w402 -> [w421 w460]
                tunnel: w401 -> [w420 w465]
                tunnel: w400 -> [w418 w466]
                tunnel: w399 -> [w423 w469]
                tunnel: w398 -> [w417 w468]
                tunnel: w397 -> [w419 w464]
                tunnel: w396 -> [w416 w463]
                frame False {
                  w425 = u16 2 items=["disabled", "Var1", "Var2", "Var1'", "Constant"] ("Function")
                  n162 = local read "Function 3"() -> (w424:u16)
                  n163 = Equal?(x=w424, y=w425) -> (x = y?=w422:bool)
                  n164 = case shown="False" w422 {
                    tunnel: w423 -> [w431 w457]
                    tunnel: w421 -> [w430 w454]
                    tunnel: w420 -> [w428 w452]
                    tunnel: w419 -> [w429 w453]
                    tunnel: w418 -> [w426 w450]
                    tunnel: w417 -> [w432 w456]
                    tunnel: w416 -> [w427 w448]
                    frame False {
                      w435 = u16 2 items=["disabled", "Var1", "Var2", "Var1'", "Constant"] ("Function")
                      n165 = local read "Function 4"() -> (w434:u16)
                      n166 = Equal?(x=w434, y=w435) -> (x = y?=w433:bool)
                      n167 = case shown="True" w433 {
                        tunnel: w432 -> [w436 w447]
                        tunnel: w431 -> [_ w446]
                        tunnel: w430 -> [_ w443]
                        tunnel: w429 -> [_ w444]
                        tunnel: w428 -> [_ w442]
                        tunnel: w427 -> [_ w438]
                        tunnel: w426 -> [_ w439]
                        frame False {
                          n168 = local write "error?"(w436) -> ()
                        }
                        frame True {
                          n169 = local read "Mode 4"() -> (w441:u16)
                          n170 = call "compliancevi3subvi.vi"("compliance (A)"=w443, "start"=w439, "compliance (V)"=w442, "total points"=w444, "step"=w438, "Mode"=w441) -> ("total points 2"=w440:u16, "compliance"=w437:dbl)  [unwired: 1 in, 1 out]
                          n171 = call "HP415xA _Config-Sweep-Secondary Sour.vi"("compliance"=w437, "step"=w438, "error in (no error)"=w447, "total points"=w440, "start"=w439, "VISA session"=w446) -> ("error out"=w445:errorcluster)  [unwired: 1 in]
                          n172 = local write "error?"(w445) -> ()
                        }
                      }
                    }
                    frame True {
                      n173 = local read "Mode 3"() -> (w458:u16)
                      n174 = call "compliancevi3subvi.vi"("compliance (A)"=w454, "start"=w450, "compliance (V)"=w452, "total points"=w453, "step"=w448, "Mode"=w458) -> ("total points 2"=w451:u16, "compliance"=w449:dbl)  [unwired: 1 in, 1 out]
                      n175 = call "HP415xA _Config-Sweep-Secondary Sour.vi"("compliance"=w449, "step"=w448, "error in (no error)"=w456, "total points"=w451, "start"=w450, "VISA session"=w457) -> ("error out"=w455:errorcluster)  [unwired: 1 in]
                      n176 = local write "error?"(w455) -> ()
                    }
                  }
                }
                frame True {
                  n177 = local read "Mode"() -> (w459:u16)
                  n178 = call "compliancevi3subvi.vi"("compliance (A)"=w460, "compliance (V)"=w465, "total points"=w464, "step"=w463, "Mode"=w459) -> ("total points 2"=w461:u16, "compliance"=w462:dbl)  [unwired: 2 in, 1 out]
                  n179 = call "HP415xA _Config-Sweep-Secondary Sour.vi"("compliance"=w462, "step"=w463, "error in (no error)"=w468, "total points"=w461, "start"=w466, "VISA session"=w469) -> ("error out"=w467:errorcluster)  [unwired: 1 in]
                  n180 = local write "error?"(w467) -> ()
                }
              }
            }
          }
        }
        frame True {
          w478 = u16 2 items=["disabled", "Var1", "Var2", "Var1'", "Constant"] ("Function 2")
          n181 = local read "error?"() -> (w480:errorcluster)
          n182 = local read "Mode"() -> (w488:u16)
          n183 = local read "Function 2"() -> (w479:u16)
          n184 = call "compliancesubvi2.vi"("compliance (V)"=w487, "Mode"=w488, "compliance (A)"=w486) -> ("compliance"=w489:dbl)  [unwired: 3 in, 1 out]
          n185 = call "HP415xA _Config-Sweep-Primary Sour.vi"("step (linear only)"=w483, "stop"=w482, "start"=w481, "compliance"=w489, "error in (no error)"=w480, "sweep mode"=w484, "sweep spacing (linear: 0)"=w485, "VISA session"=w470) -> ("error out"=w471:errorcluster)  [unwired: 2 in]
          n186 = Equal?(x=w479, y=w478) -> (x = y?=w477:bool)
          n187 = case shown="True" w477 {
            tunnel: w476 -> [w495 w539]
            tunnel: w475 -> [w496 w538]
            tunnel: w474 -> [w493 w535]
            tunnel: w473 -> [w494 w537]
            tunnel: w472 -> [w492 w533]
            tunnel: w471 -> [w491 w542]
            tunnel: w470 -> [w490 w540]
            frame False {
              w499 = u16 2 items=["disabled", "Var1", "Var2", "Var1'", "Constant"] ("Function 2")
              n188 = local read "Function 3"() -> (w498:u16)
              n189 = Equal?(x=w498, y=w499) -> (x = y?=w497:bool)
              n190 = case shown="True" w497 {
                tunnel: w496 -> [w504 w522]
                tunnel: w495 -> [w505 w523]
                tunnel: w494 -> [w502 w528]
                tunnel: w493 -> [w503 w525]
                tunnel: w492 -> [w501 w524]
                tunnel: w491 -> [w506 w531]
                tunnel: w490 -> [w500 w529]
                frame False {
                  w509 = u16 2 items=["disabled", "Var1", "Var2", "Var1'", "Constant"] ("Function 2")
                  n191 = local read "Function 4"() -> (w508:u16)
                  n192 = Equal?(x=w508, y=w509) -> (x = y?=w507:bool)
                  n193 = case shown="True" w507 {
                    tunnel: w506 -> [w510 w521]
                    tunnel: w505 -> [_ w511]
                    tunnel: w504 -> [_ w512]
                    tunnel: w503 -> [_ w513]
                    tunnel: w502 -> [_ w518]
                    tunnel: w501 -> [_ w515]
                    tunnel: w500 -> [_ w519]
                    frame False {
                      n194 = local write "error?"(w510) -> ()
                    }
                    frame True {
                      n195 = local read "Mode 4"() -> (w517:u16)
                      n196 = call "compliancevi3subvi.vi"("compliance (A)"=w511, "start"=w513, "compliance (V)"=w512, "total points"=w518, "step"=w515, "Mode"=w517) -> ("total points 2"=w514:u16, "compliance"=w516:dbl)  [unwired: 1 in, 1 out]
                      n197 = call "HP415xA _Config-Sweep-Secondary Sour.vi"("compliance"=w516, "step"=w515, "error in (no error)"=w521, "total points"=w514, "start"=w513, "VISA session"=w519) -> ("error out"=w520:errorcluster)  [unwired: 1 in]
                      n198 = local write "error?"(w520) -> ()
                    }
                  }
                }
                frame True {
                  n199 = local read "Mode 3"() -> (w532:u16)
                  n200 = call "compliancevi3subvi.vi"("compliance (A)"=w523, "start"=w525, "compliance (V)"=w522, "total points"=w528, "step"=w524, "Mode"=w532) -> ("total points 2"=w527:u16, "compliance"=w526:dbl)  [unwired: 1 in, 1 out]
                  n201 = call "HP415xA _Config-Sweep-Secondary Sour.vi"("compliance"=w526, "step"=w524, "error in (no error)"=w531, "total points"=w527, "start"=w525, "VISA session"=w529) -> ("error out"=w530:errorcluster)  [unwired: 1 in]
                  n202 = local write "error?"(w530) -> ()
                }
              }
            }
            frame True {
              n203 = local read "Mode 2"() -> (w543:u16)
              n204 = call "compliancevi3subvi.vi"("compliance (A)"=w539, "start"=w535, "compliance (V)"=w538, "total points"=w537, "step"=w533, "Mode"=w543) -> ("total points 2"=w536:u16, "compliance"=w534:dbl)  [unwired: 1 in, 1 out]
              n205 = call "HP415xA _Config-Sweep-Secondary Sour.vi"("compliance"=w534, "step"=w533, "error in (no error)"=w542, "total points"=w536, "start"=w535, "VISA session"=w540) -> ("error out"=w541:errorcluster)  [unwired: 1 in]
              n206 = local write "error?"(w541) -> ()
            }
          }
        }
      }
    }
    frame #4 {
      # "This step sets the integration time."
      n207 = local read "VISA session"() -> (w544:refnum<visa-resource-name>)
      n208 = local read "error?"() -> (w548:errorcluster)
      n209 = call "HP415xA _Config-Meas-Timing.vi"("error in (no error)"=w548, "wait time parameter"="wait time parameter", "integration time"="integration time", "VISA session"=w544) -> ("error out"=w547:errorcluster)  [unwired: 2 in]
      n210 = local write "error?"(w547) -> ()
    }
    frame #5 {
      w582 = u32 1 items=["stop  ", "single  ", "single-append  ", "stress start  ", "continuous  ", "standby on  ", "standby off  ", "zero  "] ("function (stop:0)")
      w586 = u16 2 items=["disabled", "Var1", "Var2", "Var1'", "Constant"] ("Function")
      w591 = u16 1 items=["disabled", "Var1", "Var2", "Var1'", "Constant"] ("Function")
      n211 = local read "Function"() -> (w593:u16)
      n212 = local read "Function"() -> (w585:u16)
      n213 = Equal?(x=w593, y=w591) -> (x = y?=w592:bool)
      n214 = Equal?(x=w585, y=w586) -> (x = y?=w584:bool)
      n215 = case shown="False" w592 {
        tunnel: [w819 w834] -> w587
        tunnel: [w820 w833] -> _
        tunnel: w591 -> [w817 _]
        frame False {
          n216 = local read "Function 2"() -> (w821:u16)
          n217 = Equal?(x=w821, y=w817) -> (x = y?=w818:bool)
          n218 = case shown="False" w818 {
            tunnel: [w822 w832] -> w820
            tunnel: [w823 w831] -> w819
            tunnel: w817 -> [w826 _]
            frame False {
              n219 = local read "Function 3"() -> (w825:u16)
              n220 = Equal?(x=w825, y=w826) -> (x = y?=w824:bool)
              n221 = case shown="True" w824 {
                tunnel: [w828 w830] -> w823
                tunnel: [w827 w829] -> w822
                frame False {
                  n222 = local read "Vname 4"() -> (w828:string)
                  n223 = local read "Iname 4"() -> (w827:string)
                }
                frame True {
                  n224 = local read "Vname 3"() -> (w830:string)
                  n225 = local read "Iname 3"() -> (w829:string)
                }
              }
            }
            frame True {
              n226 = local read "Vname 2"() -> (w831:string)
              n227 = local read "Iname 2"() -> (w832:string)
            }
          }
        }
        frame True {
          n228 = local read "Vname"() -> (w834:string)
          n229 = local read "Iname"() -> (w833:string)
        }
      }
      n230 = case shown="False" w584 {
        tunnel: [w677 w730] -> w558
        tunnel: [w676 TRUE ("x = y?")] -> w563
        frame False {
          w680 = u16 2 items=["disabled", "Var1", "Var2", "Var1'", "Constant"] ("Function")
          n231 = local read "Function 2"() -> (w679:u16)
          n232 = Equal?(x=w679, y=w680) -> (x = y?=w678:bool)
          n233 = case shown="True" w678 {
            tunnel: [w682 w720] -> w677
            tunnel: [w681 TRUE ("x = y?")] -> w676
            frame False {
              w685 = u16 2 items=["disabled", "Var1", "Var2", "Var1'", "Constant"] ("Function")
              n234 = local read "Function 3"() -> (w684:u16)
              n235 = Equal?(x=w684, y=w685) -> (x = y?=w683:bool)
              n236 = case shown="False" w683 {
                tunnel: [w690 w710] -> w682
                tunnel: [w686 TRUE ("x = y?")] -> w681
                frame False {
                  w689 = u16 2 items=["disabled", "Var1", "Var2", "Var1'", "Constant"] ("Function")
                  n237 = local read "Function 4"() -> (w688:u16)
                  n238 = Equal?(x=w688, y=w689) -> (x = y?=w687:bool)
                  n239 = case shown="True" w687 {
                    tunnel: ["0" ("Vname 4") w700] -> w690
                    tunnel: [FALSE ("x = y?") TRUE ("x = y?")] -> w686
                    frame False {
                    }
                    frame True {
                      w694 = u16 2 items=["V", "I", "VPulse", "IPulse", "Common"] ("Mode 2")
                      w697 = u16 0 items=["V", "I", "VPulse", "IPulse", "Common"] ("Mode 2")
                      n240 = local read "Mode 4"() -> (w696:u16)
                      n241 = Equal?(x=w697, y=w696) -> (x = y?=w698:bool)
                      n242 = Equal?(x=w696, y=w694) -> (x = y?=w695:bool)
                      n243 = Or(x=w698, y=w695) -> (x .or. y?=w693:bool)
                      n244 = case shown="False" w693 {
                        tunnel: [w701 w702] -> w700
                        frame False {
                          n245 = local read "Iname 4"() -> (w701:string)
                        }
                        frame True {
                          n246 = local read "Vname 4"() -> (w702:string)
                        }
                      }
                    }
                  }
                }
                frame True {
                  w706 = u16 2 items=["V", "I", "VPulse", "IPulse", "Common"] ("Mode 2")
                  w705 = u16 0 items=["V", "I", "VPulse", "IPulse", "Common"] ("Mode 2")
                  n247 = local read "Mode 3"() -> (w704:u16)
                  n248 = Equal?(x=w705, y=w704) -> (x = y?=w708:bool)
                  n249 = Equal?(x=w704, y=w706) -> (x = y?=w707:bool)
                  n250 = Or(x=w708, y=w707) -> (x .or. y?=w703:bool)
                  n251 = case shown="False" w703 {
                    tunnel: [w711 w712] -> w710
                    frame False {
                      n252 = local read "Iname 3"() -> (w711:string)
                    }
                    frame True {
                      n253 = local read "Vname 3"() -> (w712:string)
                    }
                  }
                }
              }
            }
            frame True {
              w714 = u16 2 items=["V", "I", "VPulse", "IPulse", "Common"] ("Mode 2")
              w715 = u16 0 items=["V", "I", "VPulse", "IPulse", "Common"] ("Mode 2")
              n254 = local read "Mode 2"() -> (w716:u16)
              n255 = Equal?(x=w715, y=w716) -> (x = y?=w718:bool)
              n256 = Equal?(x=w716, y=w714) -> (x = y?=w717:bool)
              n257 = Or(x=w718, y=w717) -> (x .or. y?=w713:bool)
              n258 = case shown="True" w713 {
                tunnel: [w721 w722] -> w720
                frame False {
                  n259 = local read "Iname 2"() -> (w721:string)
                }
                frame True {
                  n260 = local read "Vname 2"() -> (w722:string)
                }
              }
            }
          }
        }
        frame True {
          w727 = u16 2 items=["V", "I", "VPulse", "IPulse", "Common"] ("Mode")
          w728 = u16 0 items=["V", "I", "VPulse", "IPulse", "Common"] ("Mode")
          n261 = local read "Mode"() -> (w726:u16)
          n262 = Equal?(x=w726, y=w728) -> (x = y?=w725:bool)
          n263 = Equal?(x=w726, y=w727) -> (x = y?=w724:bool)
          n264 = Or(x=w725, y=w724) -> (x .or. y?=w723:bool)
          n265 = case shown="True" w723 {
            tunnel: [w731 w732] -> w730
            frame False {
              n266 = local read "Iname"() -> (w731:string)
            }
            frame True {
              n267 = local read "Vname"() -> (w732:string)
            }
          }
        }
      }
      n268 = local read "error?"() -> (w574:errorcluster)
      n269 = Unbundle("Y2 axis settings") -> ("Y2 axis on/off"=w565:bool, "MINIMUM"=w579:ext, "MAXIMUM"=w578:ext, "Variable name"=w571:string, "LIN or LOG axis"=w577:string)
      n270 = local read "Var2 step settings"() -> (w589:T3)
      n271 = local read "Var1 sweep settings"() -> (w590:T4)
      n272 = local read "VISA session"() -> (w569:refnum<visa-resource-name>)
      n273 = call "Y1subvi.vi"("MAXIMUM"="MAXIMUM", "Variable name"="Y1 axis", "error in (no error)"=w574, "MINIMUM"="MINIMUM", "LIN or LOG axis"="LIN", "VISA resource name"=w569) -> ("error out"=w575:errorcluster)
      n274 = case shown="True" w565 {
        tunnel: w575 -> [w668 w675]
        tunnel: w569 -> [_ w674]
        tunnel: w579 -> [_ w673]
        tunnel: w578 -> [_ w672]
        tunnel: w571 -> [_ w671]
        tunnel: w577 -> [_ w670]
        tunnel: [w668 w669] -> w576
        frame False {
        }
        frame True {
          n275 = call "Y2subvi.vi"("MAXIMUM"=w672, "Variable name"=w671, "error in (no error)"=w675, "MINIMUM"=w673, "LIN or LOG axis"=w670, "VISA resource name"=w674) -> ("error out"=w669:errorcluster)
        }
      }
      n276 = Unbundle(w589) -> ("total points"=w588:u16)  [unwired: 4 out]
      n277 = Decrement(x=w588) -> (x-1=w564:u16)
      n278 = Unbundle(w590) -> ("start"=w561:dbl)  [unwired: 6 out]
      n279 = call "HP415xA Op-Start-Stop.vi"("error in (no error)"=w576, "function (stop:0)"=w582, "wait until finish"=TRUE, "VISA session"=w569) -> ("error out"=w581:errorcluster)  [unwired: 6 in, 1 out]
      n280 = call "HP415xA Op-Download Trace.vi"("error in (no error)"=w581, "trace (variable) name"=w587, "VISA session"=w569) -> ("error out"=w596:errorcluster, "trace"=w562:dbl[])
      n281 = call "HP415xA Op-Download Trace.vi"("error in (no error)"=w596, "trace (variable) name"="Y1 axis", "VISA session"=w569) -> ("error out"=w572:errorcluster, "trace"=w566:dbl[])
      n282 = case shown="True" w565 {
        tunnel: w572 -> [w653 w661]
        tunnel: w569 -> [_ w660]
        tunnel: w571 -> [_ w659]
        tunnel: [w653 w658] -> w570
        tunnel: w562 -> [w651 w657]
        tunnel: w566 -> [w652 w656]
        tunnel: [w650 w655] -> w549
        tunnel: [dbl[] [] ("trace") w654] -> w560
        frame False {
          n283 = Bundle("trace"=w651, "trace"=w652) -> (w650:cluster{"trace":dbl[], "trace":dbl[]})  [unwired: 1 in]
        }
        frame True {
          n284 = call "HP415xA Op-Download Trace.vi"("error in (no error)"=w661, "trace (variable) name"=w659, "VISA session"=w660) -> ("error out"=w658:errorcluster, "trace"=w654:dbl[])
          n285 = stacked-sequence {
            tunnel: w654 -> [_ w666]
            tunnel: w657 -> [w664 w665]
            tunnel: w656 -> [w663 _]
            tunnel: [w662 _] -> w655
            frame #0 {
              n286 = Bundle("trace"=w664, "trace"=w663) -> (w662:cluster{"trace":dbl[], "trace":dbl[]})  [unwired: 1 in]
            }
            frame #1 {
              n287 = Bundle("trace"=w665, "trace"=w666) -> (→"graphic display 2":cluster{"trace":dbl[], "trace":dbl[]})  [unwired: 1 in]
            }
          }
        }
      }
      "graphic display" <- w549
      n288 = case shown="True" w563 {
        tunnel: w561 -> [_ w792]
        tunnel: w566 -> [w737 w791]
        tunnel: w562 -> [w738 w789]
        tunnel: w564 -> [_ w787]
        tunnel: w564 -> [_ _]
        tunnel: w569 -> [_ w783]
        tunnel: w570 -> [_ w782]
        tunnel: [w739 w781] -> w557
        tunnel: w558 -> [_ w780]
        tunnel: w558 -> [_ w770]
        tunnel: [dbl[] [] ("trace") w779] -> w559
        tunnel: w555 -> [_ w774]
        tunnel: w554 -> [_ w773]
        tunnel: w553 -> [_ w772]
        frame False {
          n289 = Build Array(w738, w737) -> (w734:dbl[][])
          n290 = local read "error?"() -> (w739:errorcluster)
          n291 = call-poly <vilib>:"Write To Spreadsheet File.vi"("transpose? (no:F)"=TRUE ("append to file? (new file:F)"), "format (%.3f)"="%.5e", "2D data"=w734) -> ()  [unwired: 5 in, 1 out]
        }
        frame True {
          w745 = "%s"
          w776 = "\r"
          n292 = Initialize Array("") -> (w753:string[])  [unwired: 1 in]
          n293 = call "HP415xA Op-Download Trace.vi"("error in (no error)"=w782, "trace (variable) name"=w780, "VISA session"=w783) -> ("error out"=w781:errorcluster, "trace"=w779:dbl[])
          n294 = for {
            N: w787 -> [w796]
            shift-right: [w813] -> w759
            shift-left: w789 -> [w809]
            tunnel: w792 -> [w815]
            tunnel: [w814] -> _ mode=indexing
            shift-right: [w810] -> w788
            shift-left: w791 -> [w812]
            tunnel: [w811] -> w790 mode=indexing
            shift-right: [w806] -> w766
            shift-left: w779 -> [w808]
            tunnel: w770 -> [_]
            tunnel: [w800] -> w768 mode=indexing
            shift-right: [w799] -> w757
            shift-left: w753 -> [w798]
            tunnel: [w796] -> _ mode=indexing
            n295 = Search 1D Array(1D array=w809, element=w815, start index (0)=1) -> (index of element=w807:i32)
            n296 = Split 1D Array(array=w808, index=w807) -> (first subarray=w804:dbl[], second subarray=w806:dbl[])
            n297 = Array Size(array=w804) -> (size(s)=w803:i32)
            n298 = Decrement(x=w803) -> (x-1=w802:i32)
            n299 = Split 1D Array(array=w812, index=w807) -> (first subarray=w811:dbl[], second subarray=w810:dbl[])
            n300 = Split 1D Array(array=w809, index=w807) -> (first subarray=w814:dbl[], second subarray=w813:dbl[])
            n301 = Array Subset(array=w804, index=w802) -> (w805:dbl[])  [unwired: 1 in]
            n302 = Number To Exponential String(number=w805) -> (E-format string=w801:string[])  [unwired: 3 in]
            n303 = Concatenate Strings(w801) -> (w800:string)
            n304 = Build Array (concatenate)("Id", w798) -> (w799:string[])
          }
          n305 = Build Array (concatenate)(w759, w790, w788) -> (w786:dbl[][])
          n306 = Transpose 2D Array(2D array=w786) -> (transposed array=w784:dbl[][])
          n307 = Array To Spreadsheet String(array=w784, 3:"%.5e" ("format string")) -> (spreadsheet string=w771:string)  [unwired: 1 in]
          n308 = local read "Temp (K)"() -> (w741:dbl)
          n309 = Equal?(x=w741, y=0.0) -> (x = y?=w743:bool)
          n310 = case shown="True" w743 {
            tunnel: w741 -> [w794 _]
            tunnel: [w793 ""] -> w740
            frame False {
              n311 = Number To Exponential String(number=w794) -> (E-format string=w793:string)  [unwired: 3 in]
            }
            frame True {
            }
          }
          n312 = Build Array("Vd", "Id") -> (w758:string[])
          n313 = Array Size(array=w766) -> (size(s)=w767:i32)
          n314 = Decrement(x=w767) -> (x-1=w765:i32)
          n315 = Array Subset(array=w766, index=w765) -> (w764:dbl[])  [unwired: 1 in]
          n316 = Insert Into Array(array=w758, index=2, new element=w757) -> (w756:string[])
          n317 = Number To Exponential String(number=w764) -> (E-format string=w750:string[])  [unwired: 3 in]
          n318 = Build Array (concatenate)("Vg=", w768, w750) -> (w763:string[])
          n319 = Array To Spreadsheet String(array=w756, 3:w745) -> (spreadsheet string=w762:string)  [unwired: 1 in]
          n320 = Array To Spreadsheet String(array=w763, 3:w745) -> (spreadsheet string=w769:string)  [unwired: 1 in]
          n321 = Build Array("Sample Temp (K):", w740) -> (w748:string[])
          n322 = Reshape Array(w748, 1 ("start index (0)")) -> (w746:string[])
          n323 = Array To Spreadsheet String(array=w746, 3:w745) -> (spreadsheet string=w744:string)  [unwired: 1 in]
          n324 = Concatenate Strings(w774, w776, w773, w776, w772, w744, w776, w769, w762, w771, "\r") -> (w778:string)
          n325 = call <vilib>:"Write Characters To File.vi"("append to file? (new file:F)"=TRUE, "character string"=w778, "file path (dialog if empty)"="Path") -> ()  [unwired: 2 in, 1 out]
        }
      }
      n326 = Build Array(w549) -> (w550:cluster{"trace":dbl[], "trace":dbl[]}[])
      n327 = local read "Graph Cluster"() -> (w552:cluster{"Transport":cluster{dbl[], dbl[]}[]})
      n328 = Bundle By Name(cluster=w552, "Transport"=w550) -> (w551:cluster{"Transport":cluster{dbl[], dbl[]}[]})
      n329 = local write "Graph Cluster"(w551) -> ()
      n330 = case shown="True" w565 {
        tunnel: w564 -> [_ w602]
        tunnel: w563 -> [_ w603]
        tunnel: w562 -> [_ w601]
        tunnel: w561 -> [_ w600]
        tunnel: w560 -> [_ w599]
        tunnel: w559 -> [_ w598]
        tunnel: w558 -> [_ w597]
        frame False {
        }
        frame True {
          n331 = case shown="True" w603 {
            tunnel: w602 -> [_ w619]
            tunnel: w601 -> [w607 w634]
            tunnel: w600 -> [_ w633]
            tunnel: w599 -> [w608 w632]
            tunnel: w598 -> [_ w631]
            tunnel: w597 -> [_ w614]
            frame False {
              n332 = Build Array(w607, w608) -> (w606:dbl[][])
              n333 = call-poly <vilib>:"Write To Spreadsheet File.vi"("transpose? (no:F)"=TRUE, "format (%.3f)"="%.5e", "2D data"=w606) -> ()  [unwired: 5 in, 1 out]
            }
            frame True {
              n334 = for {
                N: w619 -> [_]
                shift-right: [w645] -> w630
                shift-left: w634 -> [w646]
                tunnel: w633 -> [w648]
                tunnel: [w644] -> _ mode=indexing
                shift-right: [w641] -> w628
                shift-left: w632 -> [w643]
                tunnel: [w642] -> w629 mode=indexing
                shift-right: [w638] -> w623
                shift-left: w631 -> [w639]
                tunnel: [w635] -> w620 mode=indexing
                n335 = Search 1D Array(1D array=w646, element=w648, start index (0)=1) -> (index of element=w640:i32)
                n336 = Split 1D Array(array=w646, index=w640) -> (first subarray=w644:dbl[], second subarray=w645:dbl[])
                n337 = Split 1D Array(array=w643, index=w640) -> (first subarray=w642:dbl[], second subarray=w641:dbl[])
                n338 = Split 1D Array(array=w639, index=w640) -> (first subarray=w636:dbl[], second subarray=w638:dbl[])
                n339 = Index Array(array=w636, index=1) -> (element=w635:dbl)
              }
              n340 = Build Array (concatenate)(w630, w629, w628) -> (w627:dbl[][])
              n341 = Index Array(array=w623, index=1) -> (element=w621:dbl)
              n342 = Transpose 2D Array(2D array=w627) -> (transposed array=w626:dbl[][])
              n343 = Insert Into Array(array=w620, index=w619, new element=w621) -> (w618:dbl[])
              n344 = Array To Spreadsheet String(delimiter (Tab)=",", array=w618, 3:"%.5e" ("format string")) -> (spreadsheet string=w612:string)
              n345 = Array To Spreadsheet String(delimiter (Tab)=",", array=w626, 3:"%.5e" ("format string")) -> (spreadsheet string=w610:string)
              n346 = Concatenate Strings(w614, "," ("string")) -> (w613:string)
              n347 = Concatenate Strings(w613, w612) -> (w611:string)
              n348 = Concatenate Strings(w611, w610) -> (w609:string)
              n349 = call <vilib>:"Write Characters To File.vi"("character string"=w609) -> ()  [unwired: 4 in, 1 out]
            }
          }
        }
      }
      n350 = call "HP415xA Sys-Error Query.vi"("VISA session"=w569, "error in (no error)"=w557) -> ("error out"=w594:errorcluster)  [unwired: 2 in, 1 out]
      n351 = call "HP415xA  Close.vi"("error in (no error)"=w594, "VISA session"=w569) -> ("error out"=w595:errorcluster)
      n352 = local write "error?"(w595) -> ()
    }
  }
